vi "ConfigDevice.vi"(8 "error in (no error)":errorcluster, 11 "NHRDCPower in":refnum<class "NHRDCPower.lvclass">) -> (0 "error out":errorcluster, 3 "NHRDCPower out":refnum<class "NHRDCPower.lvclass">)   [LabVIEW 2018, in "AcPwrPlugins.lvlib" / "NHRDCPower.lvclass"]
doc: "This VI configures all the properties set by the user through the INI file or the Properties Dialog box."
uses:
  NHRDCPower.lvclass
  TypeDefs/ConfigurationTypeDefinitions.ctl
  <instrlib>/NHRDCPowerModule/NHRDCPowerModule/NHRDCPowerModule.lvlib
panel:
  out "MT":u32
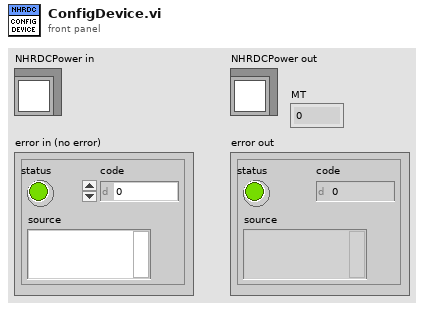
[diagram p1: front panel]
types:
  T1 = typedef "AcPwrPlugins.lvlib/NHRDCPower.lvclass/ConfigurationTypeDefinitions.ctl" = enum16{"SetWatchDog&SafetySettings", "AperatureTime", "SetRegulationGain", "Enable&SetToStandby", "UseMacros", "CleanUpPreviousMacros", "LoadMacrosFromFile", "MacroCreate&SlewRate", "MacroOperations&Delay", "MacroSave&Start", "SlewRate", "Operation"}
  T2 = typedef "AcPwrPlugins.lvlib/NHRDCPower.lvclass/Modules.ctl" = cluster{"Handle":string, "Name":string, "id query (Yes)":bool, "reset device (Yes)":bool, "Connected":bool, "Initial Battery Detect Voltage (0)":dbl, "SafetySettings":cluster{"SetWatchDog?":bool, "Voltage (V)":dbl, "Current (A)":dbl, "Power (W)":dbl, "Voltage Delay (s)":dbl, "Current Delay (s)":dbl, "Power Delay (s)":dbl}, "Options String":string, "Aperture Time (s)":dbl, "operating state (Off)":i32, "OutputSettings":cluster{"Voltage (V)":dbl, "Current (A)":dbl, "Resistance (Ohms)":dbl, "Power (W)":dbl, "Enable Voltage":bool, "Enable Current":bool, "Enable Resistance":bool, "Enable Power":bool, "Macro After Step Delay  (s)":dbl, "Wait Value (V, A, W)":dbl, "Enable Wait":bool, "Wait on Value":i32}[], "SlewRate":cluster{"Set Voltage Rate V/S":dbl, "Set Current Rate A/S":dbl, "Set Resistance Rate R/S":dbl, "Set Power Rate W/S":dbl}, "Macro":cluster{"Save Macro?":bool, "Load Macro From File?":bool, "Run Macro Continuously?":bool, "Use Macros?":bool, "Load Macro File Path":path, "Save Macro File Path":string}, "Regulation Gain (1=100%)":dbl, "UpdatingOntheFly":bool}[]
  T3 = cluster{"SetWatchDog?":bool, "Voltage (V)":dbl, "Current (A)":dbl, "Power (W)":dbl, "Voltage Delay (s)":dbl, "Current Delay (s)":dbl, "Power Delay (s)":dbl}
  T4 = cluster{"Set Voltage Rate V/S":dbl, "Set Current Rate A/S":dbl, "Set Resistance Rate R/S":dbl, "Set Power Rate W/S":dbl}
  T5 = cluster{"Voltage (V)":dbl, "Current (A)":dbl, "Resistance (Ohms)":dbl, "Power (W)":dbl, "Enable Voltage":bool, "Enable Current":bool, "Enable Resistance":bool, "Enable Power":bool, "Macro After Step Delay  (s)":dbl, "Wait Value (V, A, W)":dbl, "Enable Wait":bool, "Wait on Value":i32}[]
  T6 = cluster{"Voltage (V)":dbl, "Current (A)":dbl, "Resistance (Ohms)":dbl, "Power (W)":dbl, "Enable Voltage":bool, "Enable Current":bool, "Enable Resistance":bool, "Enable Power":bool, "Macro After Step Delay  (s)":dbl, "Wait Value (V, A, W)":dbl, "Enable Wait":bool, "Wait on Value":i32}
  T7 = cluster{"Handle":string, "Name":string, "id query (Yes)":bool, "reset device (Yes)":bool, "Connected":bool, "Initial Battery Detect Voltage (0)":dbl, "SafetySettings":cluster{"SetWatchDog?":bool, "Voltage (V)":dbl, "Current (A)":dbl, "Power (W)":dbl, "Voltage Delay (s)":dbl, "Current Delay (s)":dbl, "Power Delay (s)":dbl}, "Options String":string, "Aperture Time (s)":dbl, "operating state (Off)":i32, "OutputSettings":cluster{"Voltage (V)":dbl, "Current (A)":dbl, "Resistance (Ohms)":dbl, "Power (W)":dbl, "Enable Voltage":bool, "Enable Current":bool, "Enable Resistance":bool, "Enable Power":bool, "Macro After Step Delay  (s)":dbl, "Wait Value (V, A, W)":dbl, "Enable Wait":bool, "Wait on Value":i32}[], "SlewRate":cluster{"Set Voltage Rate V/S":dbl, "Set Current Rate A/S":dbl, "Set Resistance Rate R/S":dbl, "Set Power Rate W/S":dbl}, "Macro":cluster{"Save Macro?":bool, "Load Macro From File?":bool, "Run Macro Continuously?":bool, "Use Macros?":bool, "Load Macro File Path":path, "Save Macro File Path":string}, "Regulation Gain (1=100%)":dbl, "UpdatingOntheFly":bool}
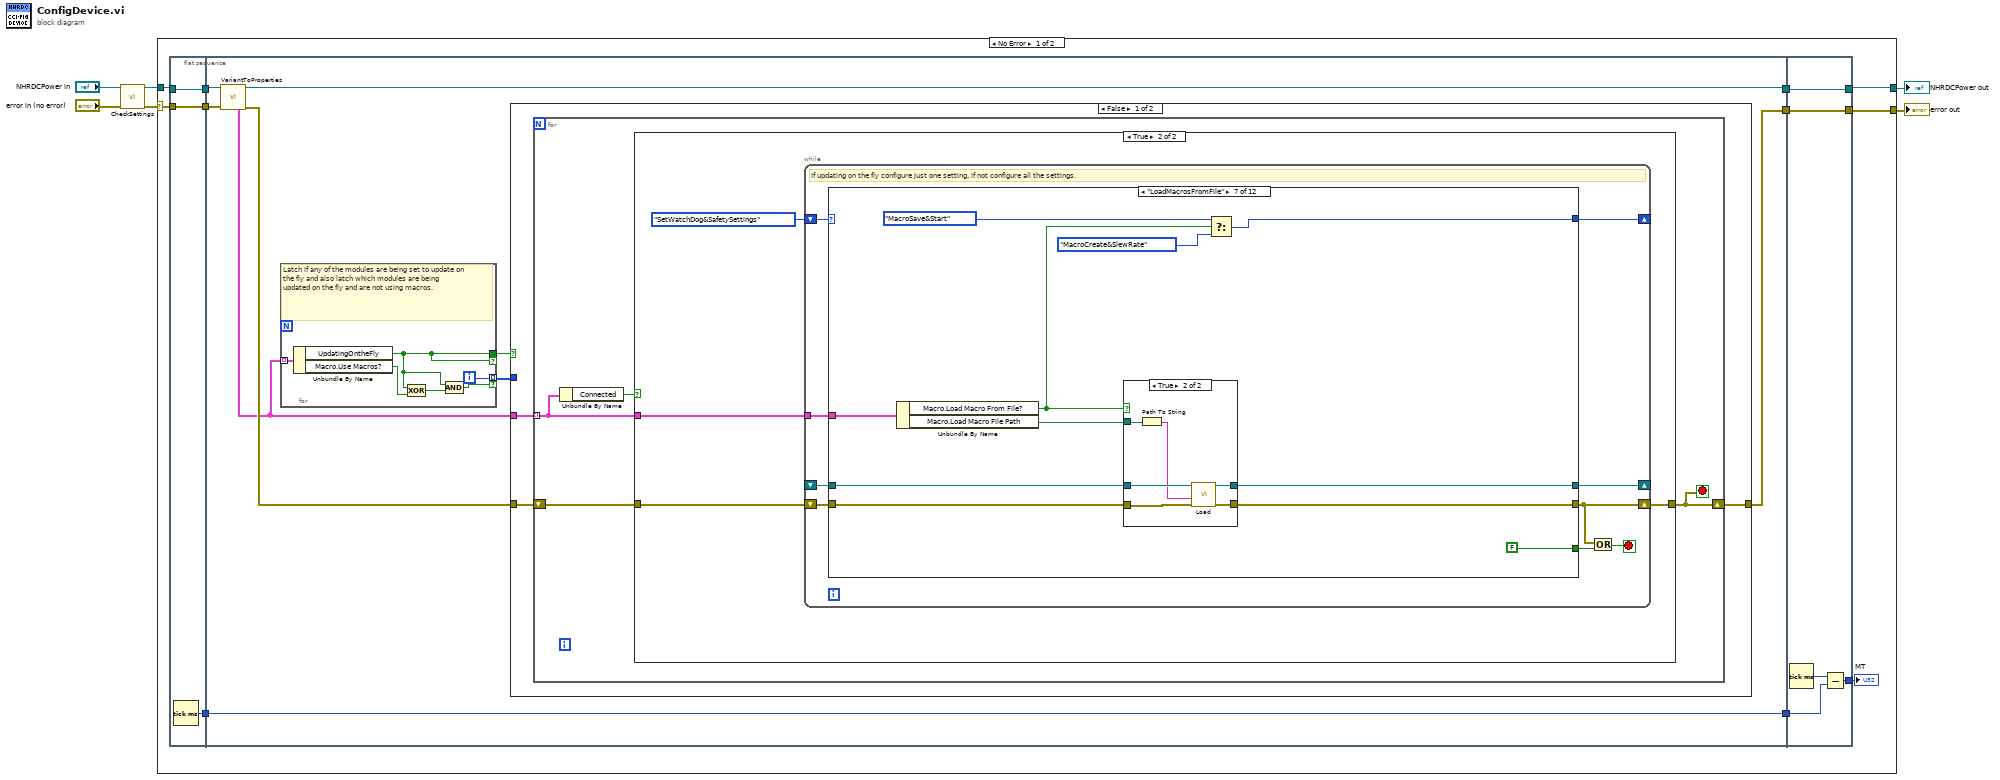
[diagram p0: block diagram]
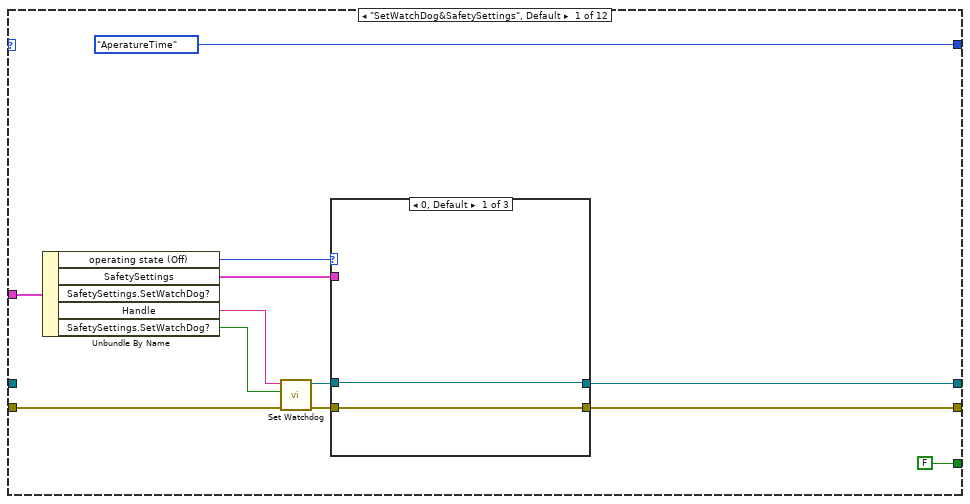
[diagram p3: hidden frame]
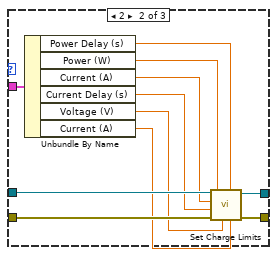
[diagram p4: hidden frame]
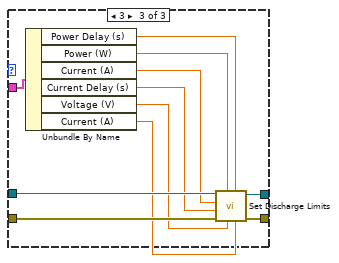
[diagram p5: hidden frame]
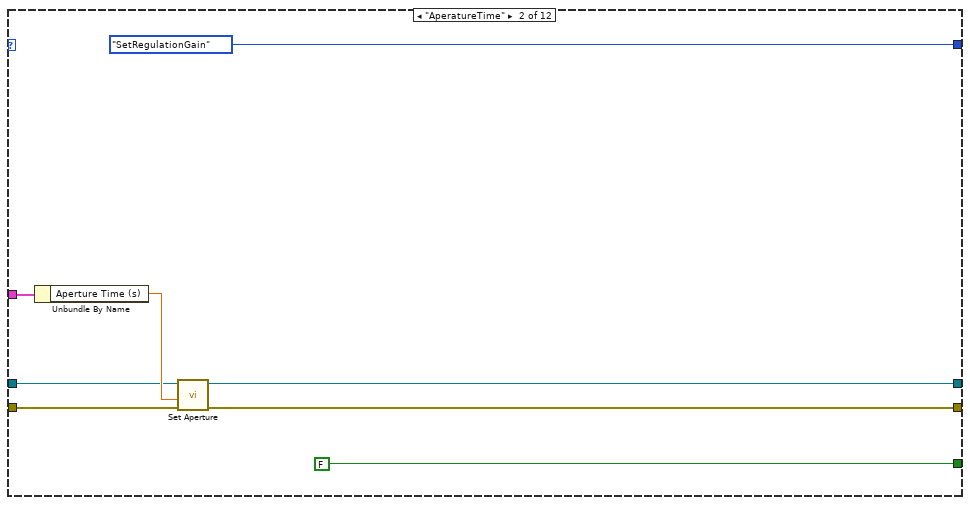
[diagram p6: hidden frame]
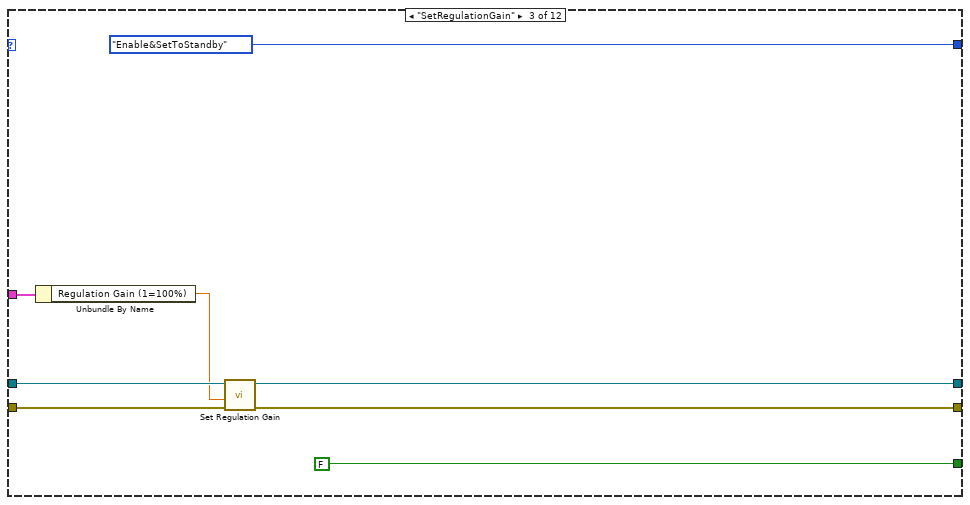
[diagram p7: hidden frame]
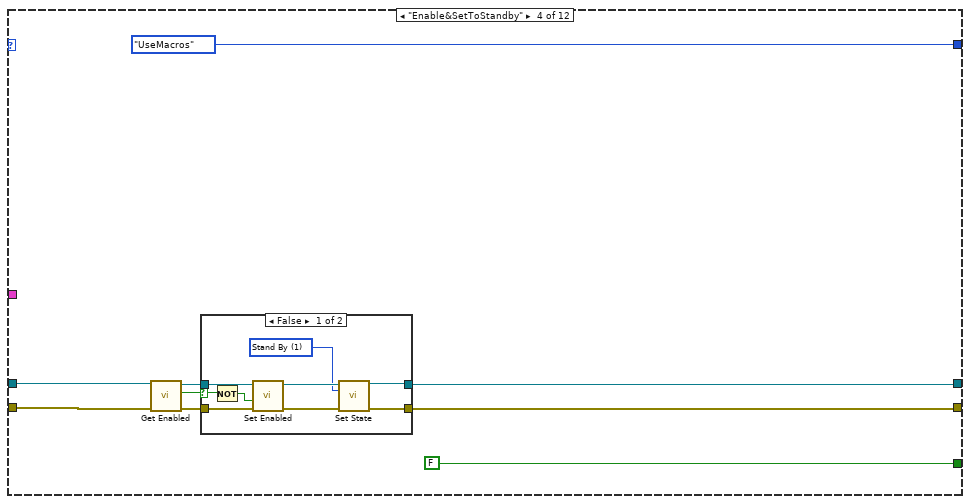
[diagram p8: hidden frame]
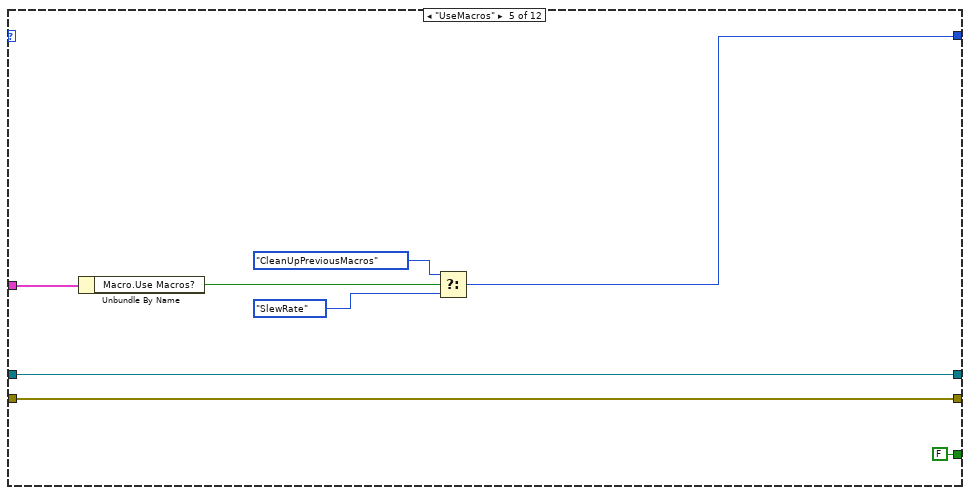
[diagram p10: hidden frame]
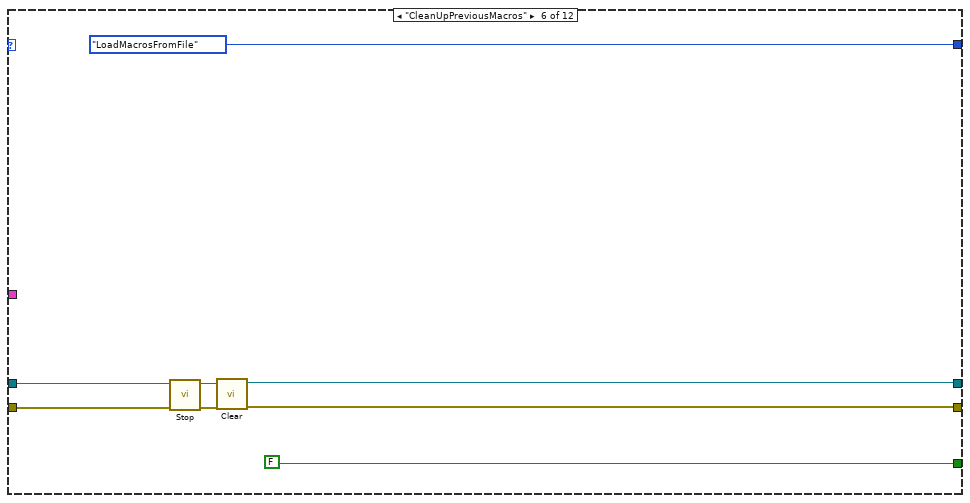
[diagram p11: hidden frame]
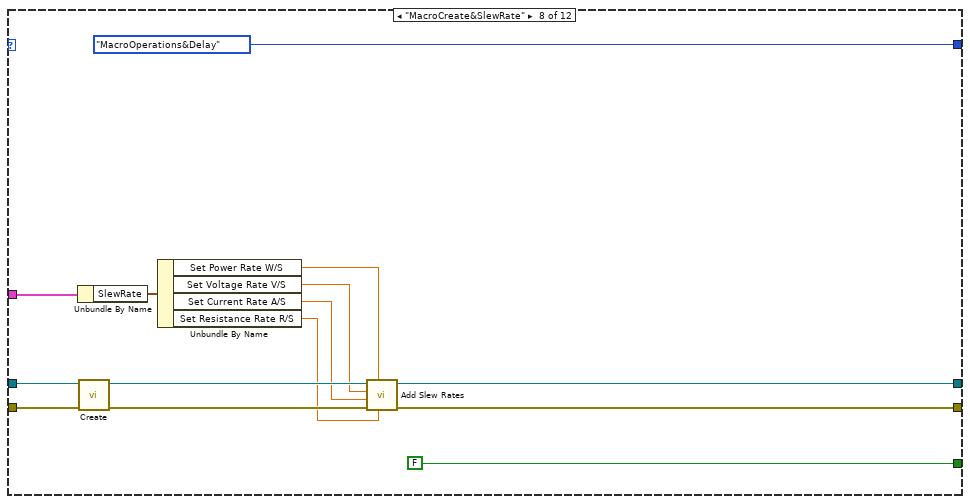
[diagram p13: hidden frame]
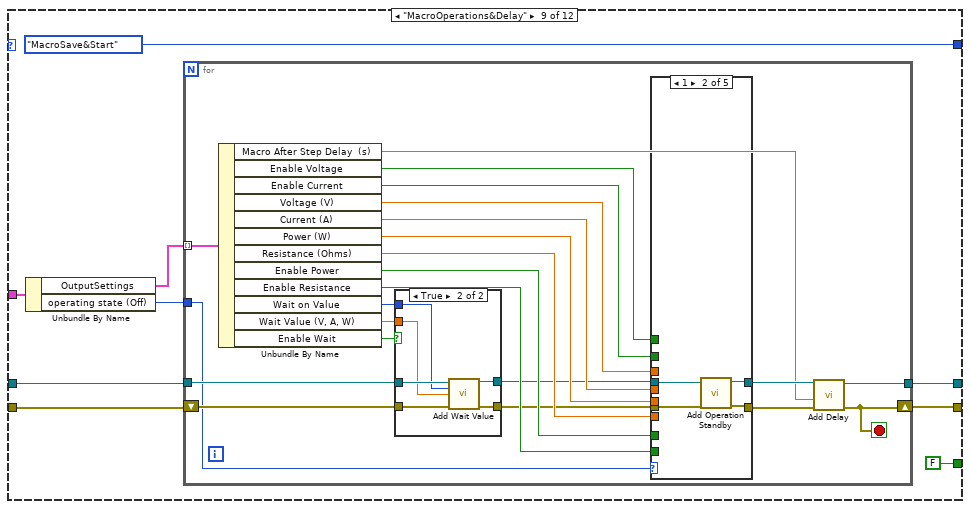
[diagram p14: hidden frame]
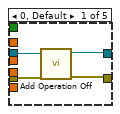
[diagram p16: hidden frame]
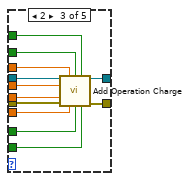
[diagram p17: hidden frame]
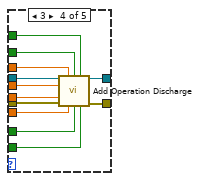
[diagram p18: hidden frame]
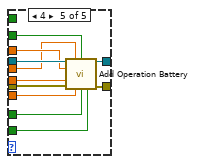
[diagram p19: hidden frame]
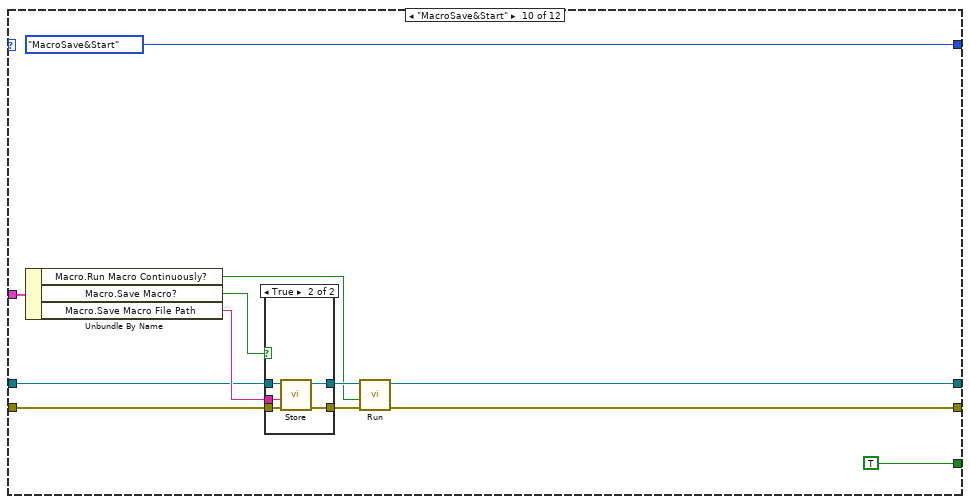
[diagram p20: hidden frame]
diagram:
  n1 = call-dynamic "CheckSettings.vi"("error in (no error)"="error in (no error)", "NHRDCPower in"="NHRDCPower in") -> ("error out"=w1:errorcluster, "NHRDCPower out"=w3:refnum<class "NHRDCPower.lvclass">)  [unwired: 8 in]
  n2 = case shown="No Error" w1 {
    selector: w1 -> [w15 w341]
    tunnel: w3 -> [w16 w342]
    tunnel: [w14 w342] -> w6
    tunnel: [w17 w341] -> w5
    frame No Error {
      n3 = flat-sequence {
        tunnel: w15 -> [w19]
        tunnel: w16 -> [w20]
        tunnel: [w20] -> w11
        tunnel: [w19] -> w10
        tunnel: [w18] -> w9
        tunnel: [w29] -> w13
        tunnel: [w26] -> w12
        tunnel: w11 -> [w28]
        tunnel: w10 -> [w27]
        tunnel: w9 -> [w21]
        tunnel: [w21] -> w8
        tunnel: [w339] -> w14
        tunnel: [w340] -> w17
        tunnel: w13 -> [w340]
        tunnel: w12 -> [w339]
        tunnel: w8 -> [w337]
        tunnel: [w336] -> w7
        frame #0 {
          n4 = Tick Count (ms)() -> (millisecond timer value=w18:u32)
        }
        frame #1 {
          n5 = call "VariantToProperties.vi"("NHRDCPower in"=w28, "error in (no error)"=w27) -> ("NHRDCPower out"=w26:refnum<class "NHRDCPower.lvclass">, "Modules"=w24:T2, "error out"=w25:errorcluster)  [unwired: 7 in, 4 out]
          n6 = for {
            tunnel: w24 -> [w335] mode=indexing
            tunnel: [w330] -> w23 if=w330
            tunnel: [w334] -> w22 mode=indexing if=w332
            i -> [w334]
            # "Latch if any of the modules are being set to update on the fly and also latch which modules are being updated on the fly and are not using macros."
            n7 = Unbundle By Name(w335) -> ("UpdatingOntheFly"=w330:bool, "Macro.Use Macros?"=w331:bool)
            n8 = Exclusive Or(1:w331, 2:w330) -> (0:w333:bool)
            n9 = And(x=w330, y=w333) -> (x .and. y?=w332:bool)
          }
          n10 = case shown="False" w23 {
            tunnel: [w32 w311] -> w29
            tunnel: w25 -> [w31 w312]
            tunnel: w24 -> [w30 w310]
            tunnel: w22 -> [_ w309]
            frame False {
              n11 = for {
                tunnel: w30 -> [w35] mode=indexing
                shift-right: [w33] -> w32
                shift-left: w31 -> [w36]
                stop <- w33 stop-if-true
                n12 = Unbundle By Name(w35) -> ("Connected"=w34:bool)
                n13 = case shown="True" w34 {
                  tunnel: w36 -> [w37 w41]
                  tunnel: [w37 w40] -> w33
                  tunnel: w35 -> [_ w39]
                  frame False {
                  }
                  frame True {
                    n14 = while {
                      tunnel: w39 -> [w48]
                      shift-right: [w47] -> w40
                      shift-left: w41 -> [w50]
                      shift-right: [w44] -> _
                      shift-left: ConfigurationTypeDefinitions."SetWatchDog&SafetySettings" ("Enum") -> [w49]
                      shift-right: [w43] -> _
                      shift-left: _ -> [w42]
                      stop <- w46 stop-if-true
                      # "If updating on the fly configure just one setting, if not configure all the settings."
                      n15 = case shown="\"LoadMacrosFromFile\"" w49 {
                        tunnel: w50 -> [w61 w94 w102 w108 w125 w134 w148 w165 w180 w262 w277 w306]
                        tunnel: w48 -> [w62 w91 w100 _ w126 _ w144 w164 w179 w265 w290 w305]
                        tunnel: [w54 w93 w98 w107 w125 w133 w146 w162 w176 w261 w275 w302] -> w47
                        tunnel: [FALSE ("x .or. y?") FALSE ("x .or. y?") FALSE ("x .or. y?") FALSE ("x .or. y?") FALSE ("x .or. y?") FALSE ("x .or. y?") FALSE ("x .or. y?") FALSE ("x .or. y?") FALSE ("x .or. y?") TRUE ("x .or. y?") FALSE ("x .or. y?") TRUE ("x .or. y?")] -> w45
                        tunnel: [ConfigurationTypeDefinitions."AperatureTime" ("Enum") ConfigurationTypeDefinitions."SetRegulationGain" ("Enum") ConfigurationTypeDefinitions."Enable&SetToStandby" ("Enum") ConfigurationTypeDefinitions."UseMacros" ("Enum") w127 ConfigurationTypeDefinitions."LoadMacrosFromFile" ("Enum") w139 ConfigurationTypeDefinitions."MacroOperations&Delay" ("Enum") ConfigurationTypeDefinitions."MacroSave&Start" ("Enum") ConfigurationTypeDefinitions."MacroSave&Start" ("Enum") ConfigurationTypeDefinitions."Operation" ("Enum") ConfigurationTypeDefinitions."Operation" ("Enum")] -> w44
                        tunnel: [w55 w88 w97 w103 w124 w132 w145 w158 w172 w254 w273 w291] -> w43
                        tunnel: w42 -> [_ w87 w96 w104 w124 w131 w147 w159 w173 w255 w274 w292]
                        frame "SetWatchDog&SafetySettings", Default {
                          n16 = Unbundle By Name(w62) -> ("operating state (Off)"=w52:i32, "SafetySettings"=w53:T3, "Handle"=w60:string, "SafetySettings.SetWatchDog?"=w51:bool)  [unwired: 1 out]
                          n17 = call <instrlib>:"Set Watchdog.vi"("error in (no error)"=w61, "watchdog"=w51, "instrument handle"=w60) -> ("error out"=w56:errorcluster, "instrument handle out"=w57:refnum<visa-resource-name>)  [unwired: 7 in]
                          n18 = case shown="0, Default" w52 {
                            tunnel: w56 -> [w64 w75 w86]
                            tunnel: [w64 w74 w85] -> w54
                            tunnel: w57 -> [w63 w73 w84]
                            tunnel: w53 -> [_ w66 w77]
                            tunnel: [w63 w65 w76] -> w55
                            frame 0, Default {
                            }
                            frame 2 {
                              n19 = Unbundle By Name(w66) -> ("Power Delay (s)"=w72:dbl, "Power (W)"=w71:dbl, "Current (A)"=w70:dbl, "Current Delay (s)"=w69:dbl, "Voltage (V)"=w68:dbl, "Current (A)"=w67:dbl)
                              n20 = call <instrlib>:"Set Charge Limits.vi"("voltage delay (0.0)"=w67, "power delay (0.0)"=w72, "voltage max"=w68, "power"=w71, "error in (no error)"=w75, "current delay (0.0)"=w69, "current"=w70, "instrument handle"=w73) -> ("error out"=w74:errorcluster, "instrument handle out"=w65:refnum<visa-resource-name>)  [unwired: 2 in]
                            }
                            frame 3 {
                              n21 = Unbundle By Name(w77) -> ("Power Delay (s)"=w83:dbl, "Power (W)"=w82:dbl, "Current (A)"=w81:dbl, "Current Delay (s)"=w80:dbl, "Voltage (V)"=w79:dbl, "Current (A)"=w78:dbl)
                              n22 = call <instrlib>:"Set Discharge Limits.vi"("voltage delay (0.0)"=w78, "power delay (0.0)"=w83, "voltage min"=w79, "power"=w82, "error in (no error)"=w86, "current delay (0.0)"=w80, "current"=w81, "instrument handle"=w84) -> ("error out"=w85:errorcluster, "instrument handle out"=w76:refnum<visa-resource-name>)  [unwired: 2 in]
                            }
                          }
                        }
                        frame "AperatureTime" {
                          n23 = Unbundle By Name(w91) -> ("Aperture Time (s)"=w89:dbl)
                          n24 = call <instrlib>:"Set Aperture.vi"("error in (no error)"=w94, "aperture (0.0)"=w89, "instrument handle"=w87) -> ("error out"=w93:errorcluster, "instrument handle out"=w88:refnum<visa-resource-name>)  [unwired: 7 in]
                        }
                        frame "SetRegulationGain" {
                          n25 = Unbundle By Name(w100) -> ("Regulation Gain (1=100%)"=w95:dbl)
                          n26 = call <instrlib>:"Set Regulation Gain.vi"("error in (no error)"=w102, "gain (0.0)"=w95, "instrument handle"=w96) -> ("error out"=w98:errorcluster, "instrument handle out"=w97:refnum<visa-resource-name>)  [unwired: 7 in]
                        }
                        frame "Enable&SetToStandby" {
                          n27 = call <instrlib>:"Get Enabled.vi"("error in (no error)"=w108, "instrument handle"=w104) -> ("error out"=w109:errorcluster, "enabled"=w111:bool, "instrument handle out"=w110:refnum<visa-resource-name>)  [unwired: 7 in]
                          n28 = case shown="False" w111 {
                            selector: w111 -> [w117 _]
                            tunnel: [w115 w121] -> w107
                            tunnel: [w113 w122] -> w103
                            tunnel: w109 -> [w119 w121]
                            tunnel: w110 -> [w118 w122]
                            frame False {
                              w112 = 1 items=["Off", "Stand By", "Charge", "Discharge", "Battery Emulation"] ("operating state (Off)")
                              n29 = Not(x=w117) -> (.not. x?=w116:bool)
                              n30 = call <instrlib>:"Set Enabled.vi"("error in (no error)"=w119, "enabled (false)"=w116, "instrument handle"=w118) -> ("error out"=w120:errorcluster, "instrument handle out"=w114:refnum<visa-resource-name>)  [unwired: 7 in]
                              n31 = call <instrlib>:"Set State.vi"("instrument handle"=w114, "operating state (Off)"=w112, "error in (no error)"=w120) -> ("instrument handle out"=w113:refnum<visa-resource-name>, "error out"=w115:errorcluster)  [unwired: 11 in]
                            }
                            frame True {
                            }
                          }
                        }
                        frame "UseMacros" {
                          n32 = Unbundle By Name(w126) -> ("Macro.Use Macros?"=w123:bool)
                          n33 = Select(t=ConfigurationTypeDefinitions."CleanUpPreviousMacros" ("Enum"), s=w123, f=ConfigurationTypeDefinitions."SlewRate" ("Enum")) -> (s? t:f=w127:T1)
                        }
                        frame "CleanUpPreviousMacros" {
                          n34 = call <instrlib>:"Stop.vi"("error in (no error)"=w134, "instrument handle"=w131) -> ("error out"=w135:errorcluster, "instrument handle out"=w136:refnum<visa-resource-name>)  [unwired: 8 in]
                          n35 = call <instrlib>:"Clear.vi"("error in (no error)"=w135, "instrument handle"=w136) -> ("error out"=w133:errorcluster, "instrument handle out"=w132:refnum<visa-resource-name>)  [unwired: 8 in]
                        }
                        frame "LoadMacrosFromFile" {
                          n36 = Unbundle By Name(w144) -> ("Macro.Load Macro From File?"=w141:bool, "Macro.Load Macro File Path"=w143:path)
                          n37 = case shown="True" w141 {
                            tunnel: w148 -> [w151 w157]
                            tunnel: [w151 w156] -> w146
                            tunnel: [w150 w155] -> w145
                            tunnel: w147 -> [w150 w154]
                            tunnel: w143 -> [_ w153]
                            frame False {
                            }
                            frame True {
                              n38 = Path To String(path=w153) -> (string=w152:string)
                              n39 = call <instrlib>:"Load.vi"("error in (no error)"=w157, "path (\"\")"=w152, "instrument handle"=w154) -> ("error out"=w156:errorcluster, "instrument handle out"=w155:refnum<visa-resource-name>)  [unwired: 7 in]
                            }
                          }
                          n40 = Select(t=ConfigurationTypeDefinitions."MacroSave&Start" ("Enum"), s=w141, f=ConfigurationTypeDefinitions."MacroCreate&SlewRate" ("Enum")) -> (s? t:f=w139:T1)
                        }
                        frame "MacroCreate&SlewRate" {
                          n41 = Unbundle By Name(w164) -> ("SlewRate"=w163:T4)
                          n42 = call <instrlib>:"Create.vi"("error in (no error)"=w165, "instrument handle"=w159) -> ("error out"=w171:errorcluster, "instrument handle out"=w170:refnum<visa-resource-name>)  [unwired: 8 in]
                          n43 = Unbundle By Name(w163) -> ("Set Power Rate W/S"=w169:dbl, "Set Voltage Rate V/S"=w168:dbl, "Set Current Rate A/S"=w167:dbl, "Set Resistance Rate R/S"=w166:dbl)
                          n44 = call <instrlib>:"Add Slew Rates.vi"("resistance slew rate (0.0)"=w166, "power slew rate (0.0)"=w169, "error in (no error)"=w171, "current slew rate (0.0)"=w167, "voltage slew rate (0.0)"=w168, "instrument handle"=w170) -> ("error out"=w162:errorcluster, "instrument handle out"=w158:refnum<visa-resource-name>)  [unwired: 4 in]
                        }
                        frame "MacroOperations&Delay" {
                          n45 = Unbundle By Name(w179) -> ("OutputSettings"=w174:T5, "operating state (Off)"=w175:i32)
                          n46 = for {
                            tunnel: w173 -> [w188]
                            shift-right: [w191] -> w176
                            shift-left: w180 -> [w190]
                            tunnel: w174 -> [w200] mode=indexing
                            tunnel: w175 -> [w185]
                            tunnel: [w181] -> w172
                            stop <- w191 stop-if-true
                            n47 = Unbundle By Name(w200) -> ("Macro After Step Delay  (s)"=w183:dbl, "Enable Voltage"=w192:bool, "Enable Current"=w193:bool, "Voltage (V)"=w194:dbl, "Current (A)"=w195:dbl, "Power (W)"=w196:dbl, "Resistance (Ohms)"=w197:dbl, "Enable Power"=w198:bool, "Enable Resistance"=w199:bool, "Wait on Value"=w184:i32, "Wait Value (V, A, W)"=w186:dbl, "Enable Wait"=w187:bool)
                            n48 = case shown="True" w187 {
                              tunnel: [w204 w210] -> w189
                              tunnel: w190 -> [w204 w209]
                              tunnel: w188 -> [w203 w208]
                              tunnel: w184 -> [_ w207]
                              tunnel: w186 -> [_ w206]
                              tunnel: [w203 w205] -> w182
                              frame False {
                              }
                              frame True {
                                n49 = call <instrlib>:"Add Wait Value.vi"("instrument handle"=w208, "wait on (Voltage Greater Than Or Equal To)"=w207, "value (0.0)"=w206, "error in (no error)"=w209) -> ("instrument handle out"=w205:refnum<visa-resource-name>, "error out"=w210:errorcluster)  [unwired: 10 in]
                              }
                            }
                            n50 = case shown="1" w185 {
                              tunnel: [w214 w218 w230 w242 w253] -> w202
                              tunnel: [w211 w215 w229 w241 w252] -> w201
                              tunnel: w189 -> [w213 w217 w228 w240 w251]
                              tunnel: w182 -> [w212 w216 w227 w239 w250]
                              tunnel: w199 -> [_ _ w226 w238 w249]
                              tunnel: w198 -> [_ _ w225 w237 w248]
                              tunnel: w197 -> [_ _ w224 w236 w243]
                              tunnel: w196 -> [_ _ w223 w235 w247]
                              tunnel: w195 -> [_ _ w222 w234 w244]
                              tunnel: w194 -> [_ _ w221 w233 w245]
                              tunnel: w193 -> [_ _ w220 w232 w246]
                              tunnel: w192 -> [_ _ w219 w231 _]
                              frame 0, Default {
                                n51 = call <instrlib>:"Add Operation Off.vi"("error in (no error)"=w213, "instrument handle"=w212) -> ("error out"=w214:errorcluster, "instrument handle out"=w211:refnum<visa-resource-name>)  [unwired: 8 in]
                              }
                              frame 1 {
                                n52 = call <instrlib>:"Add Operation Standby.vi"("error in (no error)"=w217, "instrument handle"=w216) -> ("error out"=w218:errorcluster, "instrument handle out"=w215:refnum<visa-resource-name>)  [unwired: 8 in]
                              }
                              frame 2 {
                                n53 = call <instrlib>:"Add Operation Charge.vi"("instrument handle"=w227, "voltage (0.0)"=w221, "use current (false)"=w220, "use voltage (false)"=w219, "current (0.0)"=w222, "power (0.0)"=w223, "error in (no error)"=w228, "resistance (0.0)"=w224, "use power (false)"=w225, "use resistance (false)"=w226) -> ("instrument handle out"=w229:refnum<visa-resource-name>, "error out"=w230:errorcluster)  [unwired: 4 in]
                              }
                              frame 3 {
                                n54 = call <instrlib>:"Add Operation Discharge.vi"("instrument handle"=w239, "voltage (0.0)"=w233, "use current (false)"=w232, "use voltage (false)"=w231, "current (0.0)"=w234, "power (0.0)"=w235, "error in (no error)"=w240, "resistance (0.0)"=w236, "use power (false)"=w237, "use resistance (false)"=w238) -> ("instrument handle out"=w241:refnum<visa-resource-name>, "error out"=w242:errorcluster)  [unwired: 4 in]
                              }
                              frame 4 {
                                n55 = call <instrlib>:"Add Operation Battery.vi"("instrument handle"=w250, "current (0.0)"=w244, "use current (false)"=w246, "voltage"=w245, "power (0.0)"=w247, "error in (no error)"=w251, "resistance (0.0)"=w243, "use power (false)"=w248, "use resistance (false)"=w249) -> ("instrument handle out"=w252:refnum<visa-resource-name>, "error out"=w253:errorcluster)  [unwired: 5 in]
                              }
                            }
                            n56 = call <instrlib>:"Add Delay.vi"("error in (no error)"=w202, "delay (0.0)"=w183, "instrument handle"=w201) -> ("error out"=w191:errorcluster, "instrument handle out"=w181:refnum<visa-resource-name>)  [unwired: 7 in]
                          }
                        }
                        frame "MacroSave&Start" {
                          n57 = Unbundle By Name(w265) -> ("Macro.Run Macro Continuously?"=w258:bool, "Macro.Save Macro?"=w257:bool, "Macro.Save Macro File Path"=w256:string)
                          n58 = case shown="True" w257 {
                            tunnel: w262 -> [w267 w272]
                            tunnel: [w267 w271] -> w260
                            tunnel: [w266 w270] -> w259
                            tunnel: w255 -> [w266 w269]
                            tunnel: w256 -> [_ w268]
                            frame False {
                            }
                            frame True {
                              n59 = call <instrlib>:"Store.vi"("error in (no error)"=w272, "path (\"\")"=w268, "instrument handle"=w269) -> ("error out"=w271:errorcluster, "instrument handle out"=w270:refnum<visa-resource-name>)  [unwired: 7 in]
                            }
                          }
                          n60 = call <instrlib>:"Run.vi"("error in (no error)"=w260, "continuous (false)"=w258, "instrument handle"=w259) -> ("error out"=w261:errorcluster, "instrument handle out"=w254:refnum<visa-resource-name>)  [unwired: 7 in]
                        }
                        frame "SlewRate" {
                          n61 = Unbundle By Name(w290) -> ("SlewRate"=w276:T4)
                          n62 = Unbundle By Name(w276) -> ("Set Power Rate W/S"=w278:dbl, "Set Resistance Rate R/S"=w279:dbl, "Set Current Rate A/S"=w280:dbl, "Set Voltage Rate V/S"=w281:dbl)
                          n63 = call <instrlib>:"Set Voltage Slew Rate.vi"("error in (no error)"=w277, "voltage slew rate (0.0)"=w281, "instrument handle"=w274) -> ("error out"=w287:errorcluster, "instrument handle out"=w284:refnum<visa-resource-name>)  [unwired: 7 in]
                          n64 = call <instrlib>:"Set Current Slew Rate.vi"("error in (no error)"=w287, "current slew rate (0.0)"=w280, "instrument handle"=w284) -> ("error out"=w286:errorcluster, "instrument handle out"=w283:refnum<visa-resource-name>)  [unwired: 7 in]
                          n65 = call <instrlib>:"Set Resistance Slew Rate.vi"("error in (no error)"=w286, "resistance slew rate (0.0)"=w279, "instrument handle"=w283) -> ("error out"=w285:errorcluster, "instrument handle out"=w282:refnum<visa-resource-name>)  [unwired: 7 in]
                          n66 = call <instrlib>:"Set Power Slew Rate.vi"("error in (no error)"=w285, "power slew rate (0.0)"=w278, "instrument handle"=w282) -> ("error out"=w275:errorcluster, "instrument handle out"=w273:refnum<visa-resource-name>)  [unwired: 7 in]
                        }
                        frame "Operation" {
                          n67 = Unbundle By Name(w305) -> ("OutputSettings"=w303:T5, "operating state (Off)"=w293:i32)
                          n68 = Index Array(array=w303) -> (element=w304:T6)  [unwired: 1 in]
                          n69 = Unbundle By Name(w304) -> ("Enable Voltage"=w294:bool, "Enable Current"=w295:bool, "Voltage (V)"=w296:dbl, "Current (A)"=w297:dbl, "Power (W)"=w298:dbl, "Resistance (Ohms)"=w299:dbl, "Enable Power"=w300:bool, "Enable Resistance"=w301:bool)
                          n70 = call <instrlib>:"Set State.vi"("instrument handle"=w292, "voltage (0.0)"=w296, "current enabled (false)"=w295, "voltage enabled (false)"=w294, "operating state (Off)"=w293, "current (0.0)"=w297, "power (0.0)"=w298, "error in (no error)"=w306, "resistance (0.0)"=w299, "power enabled (false)"=w300, "resistance enabled (false)"=w301) -> ("instrument handle out"=w291:refnum<visa-resource-name>, "error out"=w302:errorcluster)  [unwired: 3 in]
                        }
                      }
                      n71 = Or(x=w47, y=w45) -> (x .or. y?=w46:bool)
                    }
                  }
                }
              }
            }
            frame True {
              n72 = for {
                tunnel: w310 -> [w327]
                shift-right: [w328] -> w311
                shift-left: w312 -> [w329]
                tunnel: w309 -> [w313] mode=indexing
                # "Only update the modules which are not macros."
                n73 = Index Array(array=w327, index=w313) -> (element=w326:T7)
                n74 = Unbundle By Name(w326) -> ("OutputSettings"=w324:T5, "Handle"=w314:string, "operating state (Off)"=w315:i32)
                n75 = Index Array(array=w324) -> (element=w325:T6)  [unwired: 1 in]
                n76 = Unbundle By Name(w325) -> ("Enable Voltage"=w316:bool, "Enable Current"=w317:bool, "Voltage (V)"=w318:dbl, "Current (A)"=w319:dbl, "Power (W)"=w320:dbl, "Resistance (Ohms)"=w321:dbl, "Enable Power"=w322:bool, "Enable Resistance"=w323:bool)
                n77 = call <instrlib>:"Set State.vi"("instrument handle"=w314, "voltage (0.0)"=w318, "current enabled (false)"=w317, "voltage enabled (false)"=w316, "operating state (Off)"=w315, "current (0.0)"=w319, "power (0.0)"=w320, "error in (no error)"=w329, "resistance (0.0)"=w321, "power enabled (false)"=w322, "resistance enabled (false)"=w323) -> ("error out"=w328:errorcluster)  [unwired: 3 in, 1 out]
              }
            }
          }
        }
        frame #2 {
          n78 = Tick Count (ms)() -> (millisecond timer value=w338:u32)
          n79 = Subtract(x=w338, y=w337) -> (x-y=w336:u32)
        }
      }
      "MT" <- w7
    }
    frame Error {
    }
  }
  "error out" <- w5
  "NHRDCPower out" <- w6
